vi "FindDuplicateIssues.vi"(6 "pattern":string="*.cbz", 8 "error in":errorcluster, 11 "path":path) -> (0 "error out":errorcluster, 2 "dups found":bool, 3 "path out":path)   [LabVIEW 2024]
uses:
  <userlib>/_OpenG.lib/file/file.llb/Strip Path Extension - String__ogtk.vi
  <userlib>/_OpenG.lib/array/array.llb/Remove Duplicates from 1D Array (String)__ogtk.vi
  <userlib>/_OpenG.lib/file/file.llb/openg_file.lvlib
  <userlib>/_OpenG.lib/array/array.llb/openg_array.lvlib
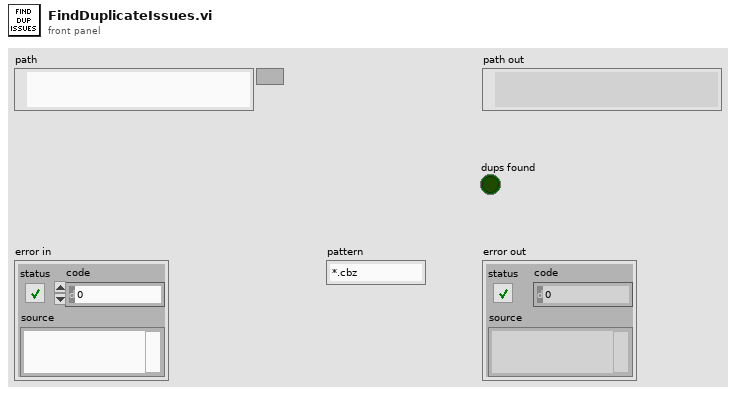
[diagram p1: front panel]
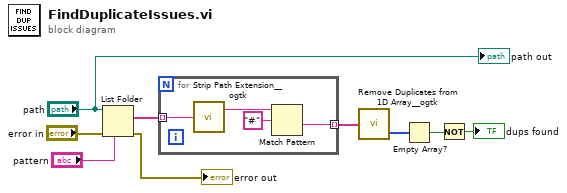
[diagram p0: block diagram]
diagram:
  n1 = List Folder(path="path", pattern="pattern", error in="error in") -> (filenames=w6:string[], error out=→"error out":errorcluster)  [unwired: 1 in, 2 out]
  n2 = for {
    tunnel: w6 -> [w13] mode=indexing
    tunnel: [w10] -> w8 mode=indexing
    n3 = call-poly <userlib>:"Strip Path Extension__ogtk.vi"("path"=w13) -> ("root"=w12:string)  [unwired: 1 out]
    n4 = Match Pattern(string=w12, regular expression="#") -> (after substring=w10:string)  [unwired: 1 in, 3 out]
  }
  n5 = call-poly <userlib>:"Remove Duplicates from 1D Array__ogtk.vi"("Input Array"=w8) -> ("indices of removed elements"=w5:i32[])  [unwired: 1 out]
  n6 = Empty Array?(array=w5) -> (empty?=w4:bool)
  n7 = Not(x=w4) -> (.not. x?=→"dups found":bool)
  "path out" <- "path"
